vi "Streaming 2945 2955 (FPGA).vi"() -> ()   [LabVIEW 2021]
doc: "Acquires data from the Rx ports and streams the data to the host while receiving data from the host and generating the resulting waveform at the Tx ports of the NI USRP 294x/295x device. Use this VI as a template for the Simple NI-USRP Streaming sample project."
uses:
  <instrlib>/_niInstr/Register Bus/v1/FPGA/Public/Read Cmd Data.ctl
  SubVIs/Stream Control State.ctl
  SubVIs/Rx Parameters 2945 2955.ctl
  Host/SubVIs/Start Trigger.ctl
  SubVIs/DDC Parameters 2945 2955.ctl
  <instrlib>/_niInstr/DSP/v1/Shared/Public/IQ Impairments.ctl
  <instrlib>/_niInstr/DSP/v1/Shared/Public/IQ Gain.ctl
  <vilib>/Platform/TimedLoop/XDataNode/timing_clust.ctl
  <vilib>/Platform/TimedLoop/XDataNode/nitl_modes.ctl
  <vilib>/Platform/TimedLoop/XDataNode/wakeup.ctl
  SubVIs/Tx Parameters.ctl
  SubVIs/DUC Parameters.ctl
  <vilib>/rvi/Emulation/niFpgaSctlEmulationGetInTimedLoop.vi
  <vilib>/rvi/Emulation/niFpgaEmulationReportErrorSimple.vi
  <vilib>/rvi/Emulation/niFpgaGetClockAttributes.vi
  <vilib>/rvi/Emulation/niFpgaCriticalErrorInLSC.vi
  <vilib>/rvi/Emulation/niFpgaProcessEmulError.vi
  <vilib>/rvi/interface/RandomDataEmulation/niFpgaRandomDataHandleErrors.vi
  <vilib>/Platform/TimedLoop/XDataNode/XDataNode.xnode
  <vilib>/rvi/DataTransferAndStorage/Container/XNode/niFpgaContainer.xnode
  <vilib>/rvi/interface/RandomDataEmulation/nirviRandomDataFpgaReadWriteTemplate.vi
  <vilib>/Platform/TimedLoop/XDataNode/XDNodeRunTimeDep.lvlib
  <instrlib>/niUsrpRio/Config/v1/FPGA/niUsrpRio Config v1 FPGA.lvlib
  <instrlib>/_niInstr/DSP/v1/Shared/niInstr DSP v1 Shared.lvlib
  <instrlib>/_niInstr/Register Bus/v1/FPGA/niInstr Register Bus v1 FPGA.lvlib
panel:
  in  "rx 3.if frequency shift":fxp<+/-,48,0> format="%#.48g"
  in  "rx 2.if frequency shift":fxp<+/-,48,0> format="%#.48g"
  in  "rx 1.if frequency shift":fxp<+/-,48,0> format="%#.48g"
  in  "rx 0.if frequency shift":fxp<+/-,48,0> format="%#.48g"
  in  "tx 1.led":enum16{"None", "RF 0/TX 1", "RF 1/TX 1"}(ring)
  in  "tx 0.led":enum16{"None", "RF 0/TX 1", "RF 1/TX 1"}(ring)
  in  "rx 0.led":T1(ring)
  in  "rx 1.led":T1(ring)
  in  "rx 2.led":T1(ring)
  in  "rx 3.led":T1(ring)
  in  "tx.data source":enum16{"SFP Port 0", "SFP Port 1", "Host"}(ring)=enum."Host"
  in  "tx.trigger sync enable":bool
  out "tx 1.number of iq data overflows":u64
  out "tx.dsp reset done":bool
  out "tx.state":T2
  out "tx 0.number of iq data overflows":u64
  out "tx.number of fifo underflows":u32
  out "tx.samples processed":u32
  in  "tx.trigger enable":bool
  in  "tx.software trigger":bool
  in  "tx.trigger select":T3=enum."Immediate"
  in  "tx 1.stream enable":bool
  in  "tx 0.stream enable":bool
  in  "tx.samples to generate":u32
  in  "tx.reset":bool=TRUE
  in  "tx.abort":bool
  in  "tx 1.gain":T4={"gain I"=1.0, "gain Q"=1.0}
  in  "tx 1.phase":fxp<+/-,21,0>
  in  "tx 1.frequency shift":fxp<+/-,48,0> format="%#.48g"
  in  "tx 1.impairments":T5={"inline gain I"=0.9999923706054688, "inline gain Q"=0.9999923706054688, "cross gain I"=0.0, "cross gain Q"=0.0, "pre-gain offset I"=0.0, "pre-gain offset Q"=0.0, "post-gain offset I"=0.0, "post-gain offset Q"=0.0}
  in  "tx 0.gain":T4={"gain I"=1.0, "gain Q"=1.0}
  in  "tx 0.impairments":T5={"inline gain I"=0.9999923706054688, "inline gain Q"=0.9999923706054688, "cross gain I"=0.0, "cross gain Q"=0.0, "pre-gain offset I"=0.0, "pre-gain offset Q"=0.0, "post-gain offset I"=0.0, "post-gain offset Q"=0.0}
  in  "tx 0.phase":fxp<+/-,21,0>
  in  "tx 0.frequency shift":fxp<+/-,48,0> format="%#.48g"
  in  "tx.delay":fxp<+/-,18,0>
  in  "tx.input sample rate":fxp<+,48,1>
  out "rx.status":T6={"rx.state"=enum."Idle", "rx.samples processed"=0, "rx.number of fifo overflows"=0, "rx.number of iq data overflows"=[0, 0, 0, 0], "rx.dsp reset done"=FALSE}
  in  "rx 2.stream enable":bool
  in  "rx 3.stream enable":bool
  out "rx 3.number of iq data overflows":u64
  out "rx 2.number of iq data overflows":u64
  in  "rx 3.impairments":T5={"inline gain I"=0.9999923706054688, "inline gain Q"=0.9999923706054688, "cross gain I"=0.0, "cross gain Q"=0.0, "pre-gain offset I"=0.0, "pre-gain offset Q"=0.0, "post-gain offset I"=0.0, "post-gain offset Q"=0.0}
  in  "rx 3.frequency shift":fxp<+/-,48,0> format="%#.48g"
  in  "rx 3.phase":fxp<+/-,21,0>
  in  "rx 2.impairments":T5={"inline gain I"=0.9999923706054688, "inline gain Q"=0.9999923706054688, "cross gain I"=0.0, "cross gain Q"=0.0, "pre-gain offset I"=0.0, "pre-gain offset Q"=0.0, "post-gain offset I"=0.0, "post-gain offset Q"=0.0}
  in  "rx 2.frequency shift":fxp<+/-,48,0> format="%#.48g"
  in  "rx 2.phase":fxp<+/-,21,0>
  in  "RF 1/Tx/Enable":bool
  in  "RF 1/Rx/Enable":bool
  in  "RF 0/Tx/Enable":bool
  in  "RF 0/Rx/Enable":bool
  in  "rx.output sample rate":fxp<+,48,1>
  in  "rx.delay":fxp<+/-,16,0>
  in  "rx 0.frequency shift":fxp<+/-,48,0> format="%#.48g"
  in  "rx 0.phase":fxp<+/-,21,0>
  in  "rx 0.impairments":T5={"inline gain I"=0.9999923706054688, "inline gain Q"=0.9999923706054688, "cross gain I"=0.0, "cross gain Q"=0.0, "pre-gain offset I"=0.0, "pre-gain offset Q"=0.0, "post-gain offset I"=0.0, "post-gain offset Q"=0.0}
  in  "rx 1.impairments":T5={"inline gain I"=0.9999923706054688, "inline gain Q"=0.9999923706054688, "cross gain I"=0.0, "cross gain Q"=0.0, "pre-gain offset I"=0.0, "pre-gain offset Q"=0.0, "post-gain offset I"=0.0, "post-gain offset Q"=0.0}
  in  "rx 1.frequency shift":fxp<+/-,48,0> format="%#.48g"
  in  "rx 1.phase":fxp<+/-,21,0>
  in  "rx.reset":bool=TRUE
  in  "rx.samples to acquire":u32
  in  "rx.abort":bool
  in  "rx 0.stream enable":bool
  in  "rx 1.stream enable":bool
  in  "rx.trigger select":T3=enum."Immediate"
  in  "rx.software trigger":bool
  in  "rx.trigger enable":bool
  out "rx.parameters":T7={"rx.trigger select"=enum."Software", "rx.trigger enable"=FALSE, "rx.trigger sync enable"=FALSE, "rx.stream enable"=[FALSE, FALSE, FALSE, FALSE], "rx.software trigger"=FALSE, "rx.reset"=FALSE, "rx.abort"=FALSE, "rx.samples to acquire"=0, "rx.data sink"=enum."SFP Port 0", "rx.ddc parameters"=[{"output sample rate"=0.0, "delay"=0.0, "frequency shift"=0.0, "impairments"={"inline gain I"=0.0, "inline gain Q"=0.0, "cross gain I"=0.0, "cross gain Q"=0.0, "pre-gain offset I"=0.0, "pre-gain offset Q"=0.0, "post-gain offset I"=0.0, "post-gain offset Q"=0.0}, "phase"=0.0, "if frequency shift"=0.0}, {"output sample rate"=0.0, "delay"=0.0, "frequency shift"=0.0, "impairments"={"inline gain I"=0.0, "inline gain Q"=0.0, "cross gain I"=0.0, "cross gain Q"=0.0, "pre-gain offset I"=0.0, "pre-gain offset Q"=0.0, "post-gain offset I"=0.0, "post-gain offset Q"=0.0}, "phase"=0.0, "if frequency shift"=0.0}, {"output sample rate"=0.0, "delay"=0.0, "frequency shift"=0.0, "impairments"={"inline gain I"=0.0, "inline gain Q"=0.0, "cross gain I"=0.0, "cross gain Q"=0.0, "pre-gain offset I"=0.0, "pre-gain offset Q"=0.0, "post-gain offset I"=0.0, "post-gain offset Q"=0.0}, "phase"=0.0, "if frequency shift"=0.0}, {"output sample rate"=0.0, "delay"=0.0, "frequency shift"=0.0, "impairments"={"inline gain I"=0.0, "inline gain Q"=0.0, "cross gain I"=0.0, "cross gain Q"=0.0, "pre-gain offset I"=0.0, "pre-gain offset Q"=0.0, "post-gain offset I"=0.0, "post-gain offset Q"=0.0}, "phase"=0.0, "if frequency shift"=0.0}]} {"rx.ddc parameters"."if frequency shift" format="%#.48g"; "rx.ddc parameters"."frequency shift" format="%#.48g"}
  out "rx.samples processed":u32
  out "rx.state":T2
  out "rx 0.number of iq data overflows":u64
  out "rx.number of fifo overflows":u32
  out "rx.dsp reset done":bool
  out "rx 1.number of iq data overflows":u64
  in  "rx.trigger sync enable":bool
  in  "rx.data sink":enum16{"SFP Port 0", "SFP Port 1", "Host"}(ring)=enum."Host"
  in  "reg.host read.go rcvd 0":bool
  out "reg.notify host.go 0":bool
  in  "reg.notify host.go rcvd 0":bool
  out "reg.host read.data 0":T9
  in  "reg.reset 0":bool
  # "FPGA utilization"
  # "USRP RIO Simple Streaming FPGA"
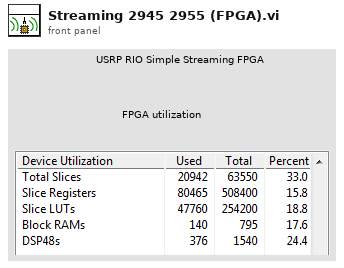
[diagram p1: front panel]
types:
  T1 = enum16{"None", "RF 0/RX 1", "RF 0/RX 2", "RF 1/RX 1", "RF 1/RX 2"}
  T2 = typedef "Stream Control State.ctl" = enum16{"Idle", "Active"}
  T3 = typedef "Start Trigger.ctl" = enum8{"Software", "Digital Edge", "Rx Start Trigger", "Tx Start Trigger", "Immediate", "Future Time Event"}
  T4 = typedef "niInstr DSP v1 Shared.lvlib/IQ Gain.ctl" = cluster{"gain I":fxp<+/-,24,3>, "gain Q":fxp<+/-,24,3>}
  T5 = typedef "niInstr DSP v1 Shared.lvlib/IQ Impairments.ctl" = cluster{"inline gain I":fxp<+/-,18,1>, "inline gain Q":fxp<+/-,18,1>, "cross gain I":fxp<+/-,18,1>, "cross gain Q":fxp<+/-,18,1>, "pre-gain offset I":fxp<+/-,18,1>, "pre-gain offset Q":fxp<+/-,18,1>, "post-gain offset I":fxp<+/-,18,1>, "post-gain offset Q":fxp<+/-,18,1>}
  T6 = cluster{"rx.state":T2, "rx.samples processed":u32, "rx.number of fifo overflows":u32, "rx.number of iq data overflows":u64[], "rx.dsp reset done":bool}
  T7 = typedef "Rx Parameters 2945 2955.ctl" = cluster{"rx.trigger select":T3, "rx.trigger enable":bool, "rx.trigger sync enable":bool, "rx.stream enable":bool[], "rx.software trigger":bool, "rx.reset":bool, "rx.abort":bool, "rx.samples to acquire":u32, "rx.data sink":enum16{"SFP Port 0", "SFP Port 1", "Host"}, "rx.ddc parameters":T8[]}
  T8 = typedef "DDC Parameters 2945 2955.ctl" = cluster{"output sample rate":fxp<+,48,1>, "delay":fxp<+/-,16,0>, "frequency shift":fxp<+/-,48,0>, "impairments":T5, "phase":fxp<+/-,21,0>, "if frequency shift":fxp<+/-,48,0>}
  T9 = typedef "niInstr Register Bus v1 FPGA.lvlib/Read Cmd Data.ctl" = cluster{"go":bool, "data":u32}
  T10 = typedef "XDNodeRunTimeDep.lvlib/timing_clust.ctl" = cluster{"Expected End [f-1]":u64, "Actual End [f-1]":u64, "Finished Late? [f-1]":bool, "Expected End [i-1]":u64, "Actual End [i-1]":u64, "Finished Late? [i-1]":bool, "Expected Start [i]":u64, "Actual Start [i]":u64, "Expected Start [f]":u64, "Actual Start [f]":u64, "Source Name":string, "Structure Name":string, "Period":i64, "Deadline":i64, "Offset":i64, "Start":i64, "Priority":i32, "Timeout":i32, "Mode":T11, "Wakeup Reason":T12, "Error":errorcluster, "Source Type":string, "Secondary Source Type":string, "Global End Time":u64, "Global Start Time":u64, "Frame Duration":u64, "Iteration Duration":u64, "Assigned CPU":i32, "I/O Scan Engine Mode":u32}
  T11 = typedef "XDNodeRunTimeDep.lvlib/nitl_modes.ctl" = enum32{"No Change", "Process missed periods, maintain original phase", "Discard missed periods, maintain original phase", "Process missed periods, ignore original phase", "Discard missed periods, ignore original phase"}
  T12 = typedef "XDNodeRunTimeDep.lvlib/wakeup.ctl" = enum32{"Normal", "Aborted", "Asynchronous wakeup", "Timing source error", "Timed loop error", "Timeout"}
  T13 = cluster{"rx 0.led":enum16{"None", "RF 0/RX 1", "RF 0/RX 2", "RF 1/RX 1", "RF 1/RX 2"}, "rx 1.led":enum16{"None", "RF 0/RX 1", "RF 0/RX 2", "RF 1/RX 1", "RF 1/RX 2"}, "rx 2.led":enum16{"None", "RF 0/RX 1", "RF 0/RX 2", "RF 1/RX 1", "RF 1/RX 2"}, "rx 3.led":enum16{"None", "RF 0/RX 1", "RF 0/RX 2", "RF 1/RX 1", "RF 1/RX 2"}}
  T14 = cluster{"rx.trigger select":T3, "rx.trigger enable":bool, "rx.trigger sync enable":bool, bool[], "rx.software trigger":bool, "rx.reset":bool, "rx.abort":bool, "rx.samples to acquire":u32, "rx.data sink":enum16{"SFP Port 0", "SFP Port 1", "Host"}, T8[]}
  T15 = cluster{"DAC FIFO Reset":refnum<k21>, "RF 0 Rx Swap IQ":refnum<k21>, "RF 0 Rx Negate I":refnum<k21>, "RF 0 Rx Negate Q":refnum<k21>, "RF 0 Rx Data Valid":refnum<k21>, "RF 0 Rx Data Ever Invalid":refnum<k21>, "clear RF 0 Rx Data Ever Invalid":refnum<k21>, "RF 0 Tx Swap IQ":refnum<k21>, "RF 0 Tx Negate I":refnum<k21>, "RF 0 Tx Negate Q":refnum<k21>, "RF 1 Rx Swap IQ":refnum<k21>, "RF 1 Rx Negate I":refnum<k21>, "RF 1 Rx Negate Q":refnum<k21>, "RF 1 Rx Data Valid":refnum<k21>, "RF 1 Rx Data Ever Invalid":refnum<k21>, "clear RF 1 Rx Data Ever Invalid":refnum<k21>, "RF 1 Tx Swap IQ":refnum<k21>, "RF 1 Tx Negate I":refnum<k21>, "RF 1 Tx Negate Q":refnum<k21>}
  T16 = typedef "niUsrpRio Synchronization v1 FPGA.lvlib/Resources.ctl" = cluster{"master":refnum<k21>, "meas.enable":refnum<k21>, "meas.ready":refnum<k21>, "meas.reset":refnum<k21>, "meas.arm":refnum<k21>, "meas.valid":refnum<k21>, "meas.value":refnum<k21>, "meas.oversample factor":refnum<k21>, "cptr":refnum<k21>, "cptr.adjust":refnum<k21>, "cptr.period":refnum<k21>}
  T17 = typedef "niUsrpRio Time v1 FPGA.lvlib/Time Resources.ctl" = cluster{"reset":refnum<k21>, "time":refnum<k21>, "time.previous cptr":refnum<k21>, "new time":refnum<k21>, "new time.when":refnum<k21>, "new time.set":refnum<k21>, "which edge of ref":refnum<k21>, "pps source":refnum<k21>, "internal pps period":refnum<k21>}
  T18 = typedef "niUsrpRio Time v1 FPGA.lvlib/Future Event Resources.ctl" = cluster{"reset":refnum<k21>, "future event.time":refnum<k21>, "future event.ready":refnum<k21>, "future event.set":refnum<k21>, "future event.clear":refnum<k21>, "future event.set in past":refnum<k21>}
  T19 = cluster{"time.resources":T17, "future event.resources":T18, "future event.resources":T18, "future event.resources":T18}
  T20 = typedef "Clock Cross Resources.ctl" = cluster{"register instruction":refnum<k21>, "read completion":refnum<k21>}
  T21 = typedef "niInstr Register Bus v1 FPGA.lvlib/Register Instruction.ctl" = cluster{"subsystem":u8, "address":u16, "data":u32, "valid":bool, "read":bool}
  T22 = typedef "niInstr Register Bus v1 FPGA.lvlib/Read Completion.ctl" = cluster{"data":u32, "valid":bool}
  T23 = typedef "Tx Parameters.ctl" = cluster{"tx.trigger select":T3, "tx.trigger enable":bool, "tx.trigger sync enable":bool, "tx.stream enable":bool[], "tx.software trigger":bool, "tx.reset":bool, "tx.abort":bool, "tx.samples to generate":u32, "tx.data source":enum16{"SFP Port 0", "SFP Port 1", "Host"}, "tx.duc parameters":T24[]}
  T24 = typedef "DUC Parameters.ctl" = cluster{"frequency shift":fxp<+/-,48,0>, "impairments":T5, "phase":fxp<+/-,21,0>, "input sample rate":fxp<+,48,1>, "gain":T4, "delay":fxp<+/-,18,0>}
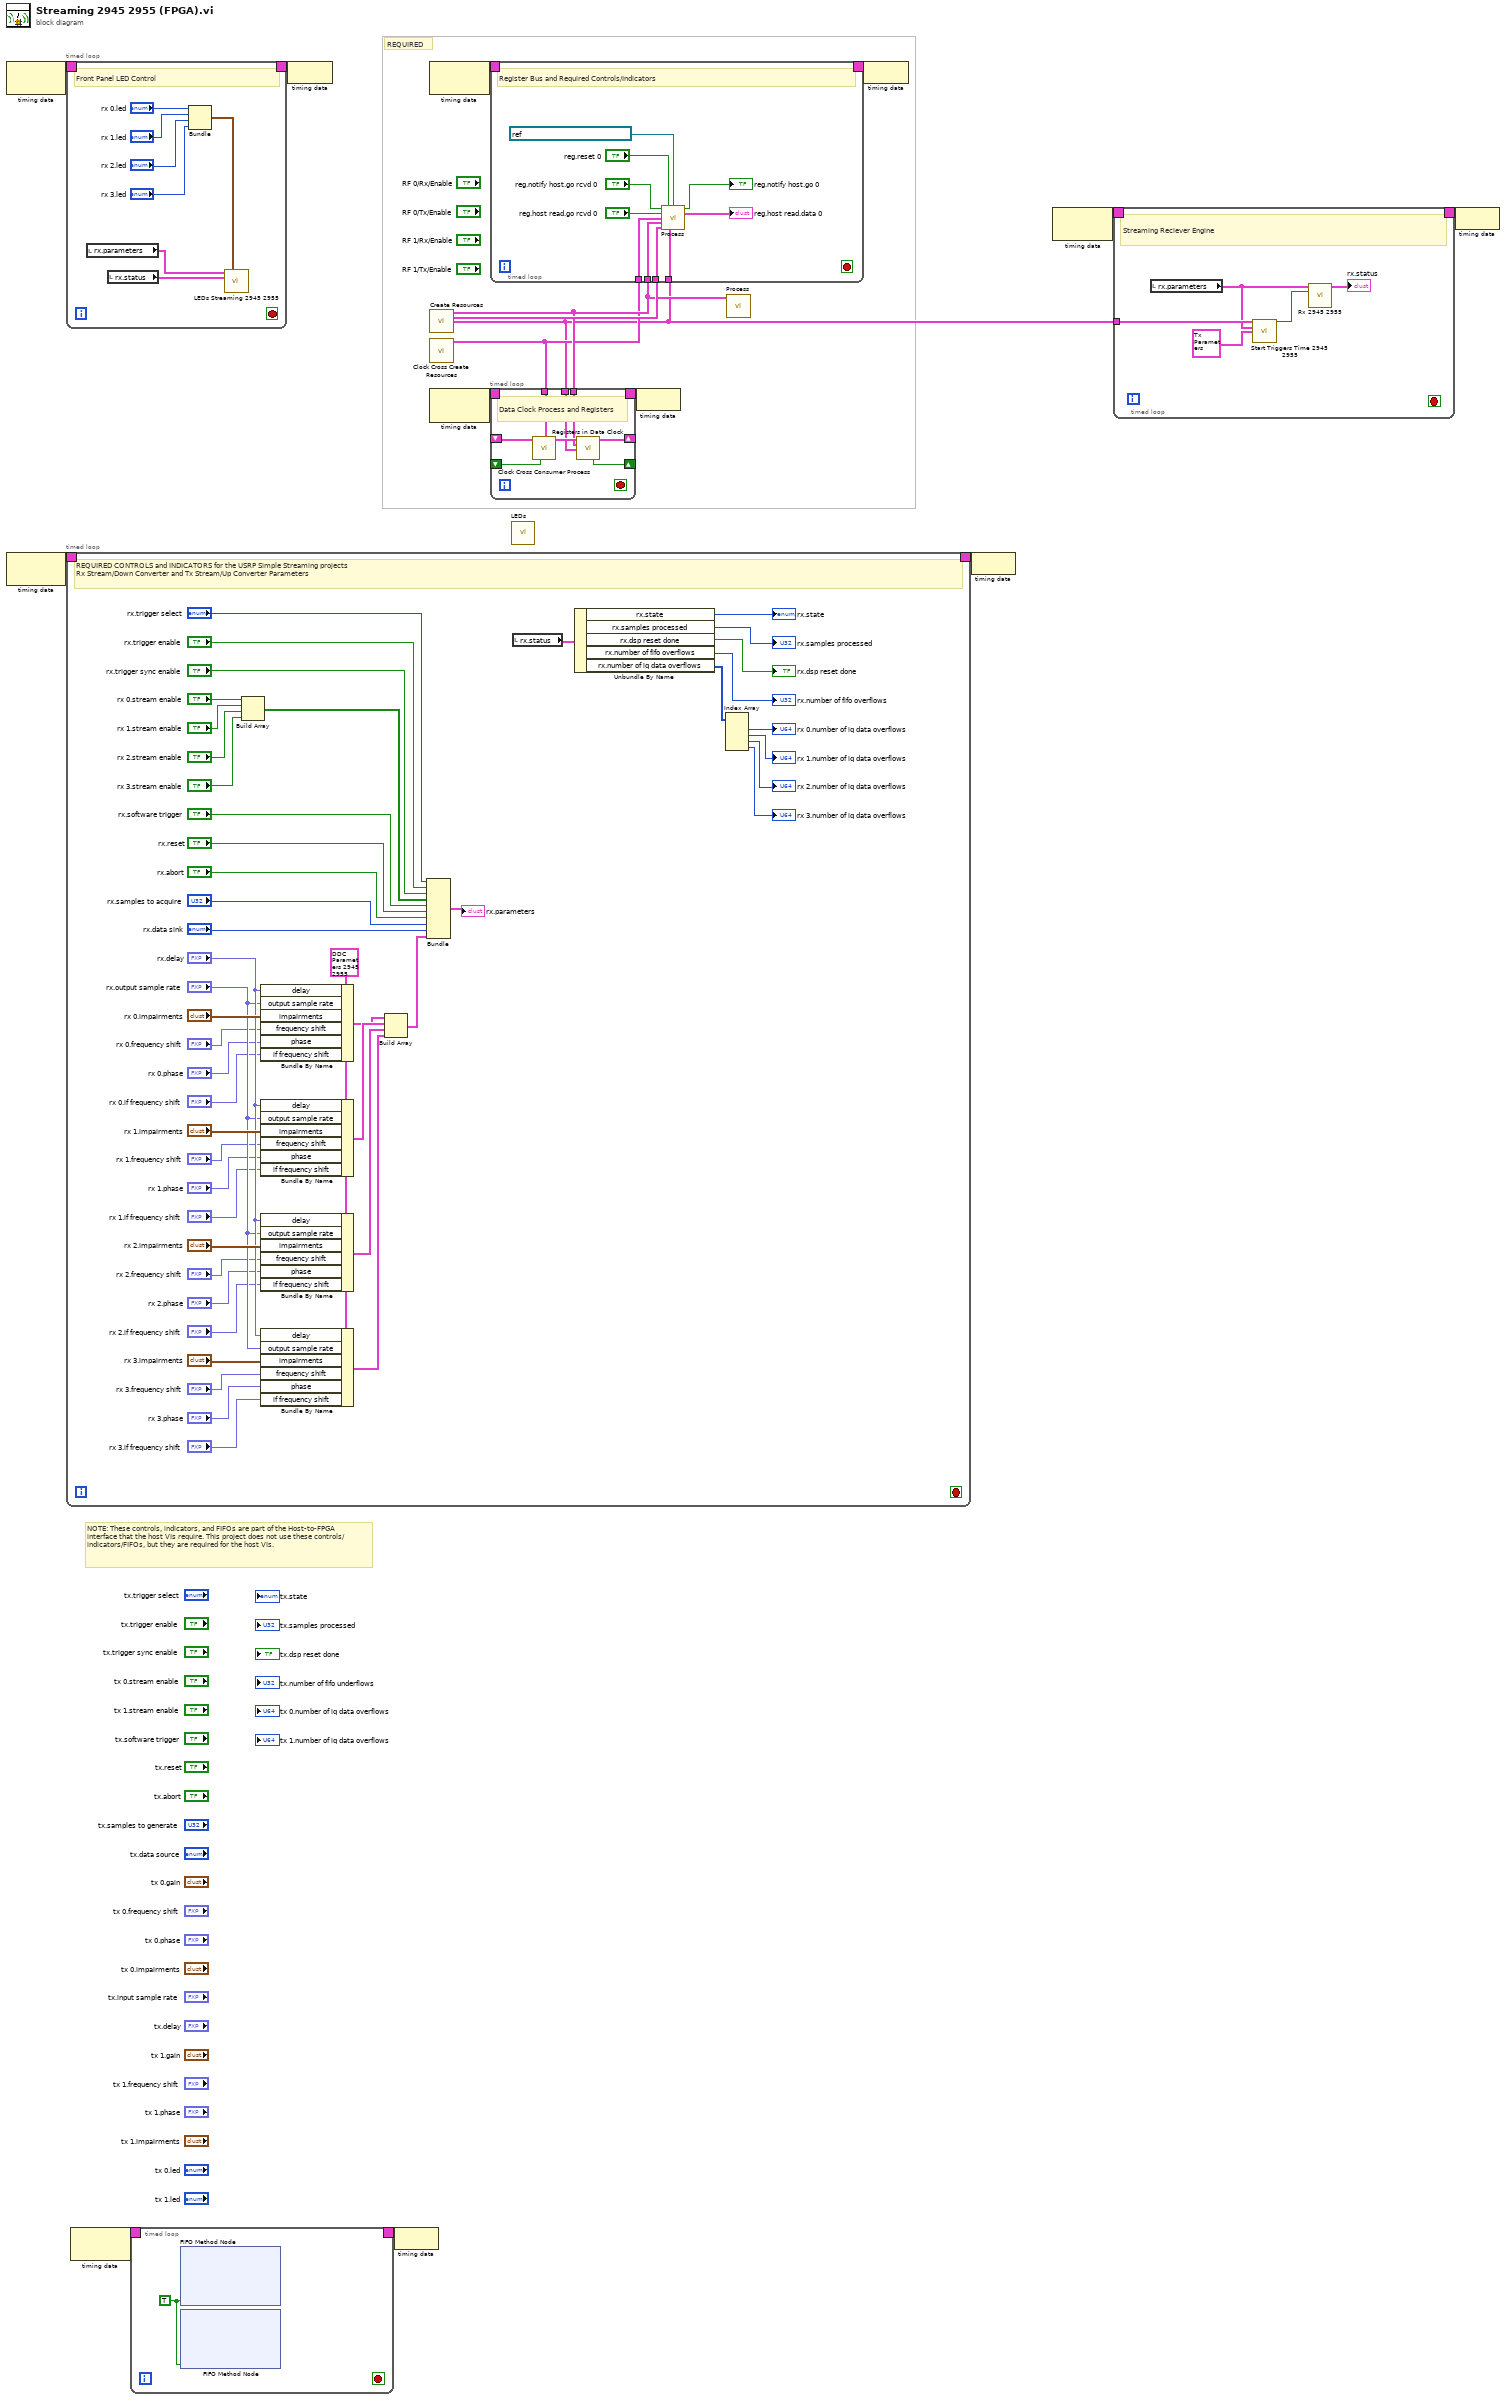
[diagram p0: block diagram]
diagram:
  # "NOTE: These controls, indicators, and FIFOs are part of the Host-to-FPGA interface that the host VIs require. This project does not use these controls/indicators/FIFOs, but they are required for the host VIs."
  # "REQUIRED"
  n1 = node-c288() -> (w2:T10)  [unwired: 1 in]
  n2 = node-c288() -> (w12:T10)  [unwired: 1 in]
  n3 = timed-loop {
    timing: w2 -> [_]
    timing-out: [_] -> w1
    stop <- _ stop-if-true
    # "Front Panel LED Control"
    n4 = local read "rx.parameters"() -> (w18:T7)
    n5 = local read "rx.status"() -> (w17:T6)
    n6 = Bundle("rx 0.led"="rx 0.led", "rx 1.led"="rx 1.led", "rx 2.led"="rx 2.led", "rx 3.led"="rx 3.led") -> (w19:T13)  [unwired: 1 in]
    n7 = call "LEDs Streaming 2945 2955.vi"("rx.parameters"=w18, "rx.leds"=w19, "rx.status"=w17) -> ()  [unwired: 13 in]
  }
  n8 = timed-loop {
    timing: w12 -> [_]
    timing-out: [_] -> w11
    stop <- _ stop-if-true
    w56 = T8 {"output sample rate"=1.0, "delay"=0.0, "frequency shift"=0.0, "impairments"={"inline gain I"=0.9999923706054688, "inline gain Q"=0.9999923706054688, "cross gain I"=0.0, "cross gain Q"=0.0, "pre-gain offset I"=0.0, "pre-gain offset Q"=0.0, "post-gain offset I"=0.0, "post-gain offset Q"=0.0}, "phase"=0.0, "if frequency shift"=0.0} ("DDC Parameters")
    # "REQUIRED CONTROLS and INDICATORS for the USRP Simple Streaming projects\nRx Stream/Down Converter and Tx Stream/Up Converter Parameters"
    n9 = Build Array("rx 0.stream enable", "rx 1.stream enable", "rx 2.stream enable", "rx 3.stream enable") -> (w37:bool[])
    n10 = Bundle By Name(cluster=w56, "delay"="rx.delay", "output sample rate"="rx.output sample rate", "impairments"="rx 0.impairments", "frequency shift"="rx 0.frequency shift", "phase"="rx 0.phase", "if frequency shift"="rx 0.if frequency shift") -> (w72:T8)
    n11 = Bundle By Name(cluster=w56, "delay"="rx.delay", "output sample rate"="rx.output sample rate", "impairments"="rx 1.impairments", "frequency shift"="rx 1.frequency shift", "phase"="rx 1.phase", "if frequency shift"="rx 1.if frequency shift") -> (w73:T8)
    n12 = Bundle By Name(cluster=w56, "delay"="rx.delay", "output sample rate"="rx.output sample rate", "impairments"="rx 2.impairments", "frequency shift"="rx 2.frequency shift", "phase"="rx 2.phase", "if frequency shift"="rx 2.if frequency shift") -> (w53:T8)
    n13 = Bundle By Name(cluster=w56, "delay"="rx.delay", "output sample rate"="rx.output sample rate", "impairments"="rx 3.impairments", "frequency shift"="rx 3.frequency shift", "phase"="rx 3.phase", "if frequency shift"="rx 3.if frequency shift") -> (w52:T8)
    n14 = Build Array(w72, w73, w53, w52) -> (w63:T8[])
    n15 = Bundle("rx.trigger select"="rx.trigger select", "rx.trigger enable"="rx.trigger enable", "rx.trigger sync enable"="rx.trigger sync enable", w37, "rx.software trigger"="rx.software trigger", "rx.reset"="rx.reset", "rx.abort"="rx.abort", "rx.samples to acquire"="rx.samples to acquire", "rx.data sink"="rx.data sink", w63) -> (→"rx.parameters":T14)  [unwired: 1 in]
    n16 = local read "rx.status"() -> (w62:T6)
    n17 = Unbundle By Name(w62) -> ("rx.state"=→"rx.state":T2, "rx.samples processed"=→"rx.samples processed":u32, "rx.dsp reset done"=→"rx.dsp reset done":bool, "rx.number of fifo overflows"=→"rx.number of fifo overflows":u32, "rx.number of iq data overflows"=w34:u64[])
    n18 = Index Array(array=w34) -> (element #1=→"rx 0.number of iq data overflows":u64, element #2=→"rx 1.number of iq data overflows":u64, element #3=→"rx 2.number of iq data overflows":u64, element #4=→"rx 3.number of iq data overflows":u64)  [unwired: 4 in]
  }
  n19 = node-c288() -> (w4:T10)  [unwired: 1 in]
  n20 = timed-loop {
    timing: w4 -> [_]
    timing-out: [_] -> w3
    stop <- _ stop-if-true
    w76 = TRUE ("Ready for Output")
    n21 = xnode ("FIFO Method Node")("Ready for Output"=w76) -> ()  [unwired: 1 in, 3 out]
    n22 = xnode ("FIFO Method Node")("Ready for Output"=w76) -> ()  [unwired: 1 in, 3 out]
  }
  n23 = node-c288(w1) -> ()
  n24 = node-c288(w3) -> ()
  n25 = node-c288() -> (w16:T10)  [unwired: 1 in]
  n26 = call "Create Resources.vi"() -> ("config.resources"=w7:T15, "sync.resources"=w10:T16, "time.resources"=w5:T19)  [unwired: 13 in]
  n27 = call "Clock Cross Create Resources.vi"() -> ("resources"=w6:T20)  [unwired: 15 in]
  n28 = node-c288() -> (w9:T10)  [unwired: 1 in]
  n29 = timed-loop "Register Bus and Required Controls/Indicators" {
    timing: w16 -> [_]
    timing-out: [_] -> w15
    tunnel: w7 -> [w81]
    tunnel: w10 -> [w80]
    tunnel: w5 -> [w79]
    tunnel: w6 -> [w82]
    stop <- _ stop-if-true
    # "Register Bus and Required Controls/Indicators"
    n30 = call <instrlib>:"Process.vi"("reg.notify host.go rcvd"="reg.notify host.go rcvd 0", "reg.reset"="reg.reset 0", "reg.instruction fifo"=refnum<k21> "reg.host instruction fifo 0" ("reg.host instruction fifo"), "reg.host read.go rcvd"="reg.host read.go rcvd 0", "clock cross resources"=w82, "config.resources"=w81, "sync.resources"=w80, "time.resources"=w79) -> ("reg.notify host.go"=→"reg.notify host.go 0":bool, "reg.host read.data"=→"reg.host read.data 0":T9)  [unwired: 6 in]
  }
  n31 = timed-loop {
    timing: w9 -> [_]
    timing-out: [_] -> w8
    shift-right: [w97] -> _
    shift-left: _ -> [w94]
    shift-right: [w96] -> _
    shift-left: _ -> [w95]
    tunnel: w7 -> [w93]
    tunnel: w6 -> [w92]
    tunnel: w5 -> [w91]
    stop <- _ stop-if-true
    # "Data Clock Process and Registers"
    n32 = call "Clock Cross Consumer Process.vi"("read completion"=w94, "resources"=w92, "ready for output"=w95) -> ("register instruction"=w98:T21)  [unwired: 12 in]
    n33 = call "Registers in Data Clock.vi"("register instruction"=w98, "config.resources"=w93, "time.resources"=w91) -> ("read completion out"=w97:T22, "ready for input"=w96:bool)  [unwired: 11 in]
  }
  n34 = call "LEDs.vi"() -> ()  [unwired: 1 in]
  n35 = node-c288(w8) -> ()
  n36 = call <instrlib>:"Process.vi"("resources"=w7) -> ()  [unwired: 15 in]
  n37 = node-c288(w15) -> ()
  n38 = node-c288(w11) -> ()
  n39 = node-c288() -> (w14:T10)  [unwired: 1 in]
  n40 = timed-loop "Streaming Transceiver Engine" {
    timing: w14 -> [_]
    timing-out: [_] -> w13
    tunnel: w5 -> [w104]
    stop <- _ stop-if-true
    # "Streaming Reciever Engine"
    n41 = local read "rx.parameters"() -> (w103:T7)
    n42 = call "Start Triggers Time 2945 2955.vi"("time.resources"=w104, "rx.parameters"=w103, "tx.parameters"=T23 {"tx.trigger select"=enum."Software", "tx.trigger enable"=FALSE, "tx.trigger sync enable"=FALSE, "tx.stream enable"=[FALSE, FALSE], "tx.software trigger"=FALSE, "tx.reset"=FALSE, "tx.abort"=FALSE, "tx.samples to generate"=0, "tx.data source"=enum."SFP Port 0", "tx.duc parameters"=[{"frequency shift"=0.0, "impairments"={"inline gain I"=0.0, "inline gain Q"=0.0, "cross gain I"=0.0, "cross gain Q"=0.0, "pre-gain offset I"=0.0, "pre-gain offset Q"=0.0, "post-gain offset I"=0.0, "post-gain offset Q"=0.0}, "phase"=0.0, "input sample rate"=0.0, "gain"={"gain I"=0.0, "gain Q"=0.0}, "delay"=0.0}, {"frequency shift"=0.0, "impairments"={"inline gain I"=0.0, "inline gain Q"=0.0, "cross gain I"=0.0, "cross gain Q"=0.0, "pre-gain offset I"=0.0, "pre-gain offset Q"=0.0, "post-gain offset I"=0.0, "post-gain offset Q"=0.0}, "phase"=0.0, "input sample rate"=0.0, "gain"={"gain I"=0.0, "gain Q"=0.0}, "delay"=0.0}]}) -> ("rx.start trigger"=w105:bool)  [unwired: 11 in, 1 out]
    n43 = call "Rx 2945 2955.vi"("rx.parameters"=w103, "rx.start trigger"=w105) -> ("rx.status"=→"rx.status":T6)  [unwired: 13 in]
  }
  n44 = node-c288(w13) -> ()
